vi "Example--SMO.Example.vi"() -> ()   [LabVIEW 2013]
uses:
  SMO.UI.Example/SMO.UI.Example.lvclass
  SMO/Typedefs/SMOState --Enum.ctl
  SMO/Protected/ListThisLevelDependencies.vi
  SMO/reuse/CastArrayDependenciesToClusterOrClass.vi
  SMO.Example/SMO.Example.lvclass
  SMO.UI/SMO.UI.lvclass
  SMO/SMO.lvclass
panel:
  in  "About":bool
  out "Data Changed":string
  out "error out":errorcluster
  in  "Stop":bool
  # "SMO Example Launcher"
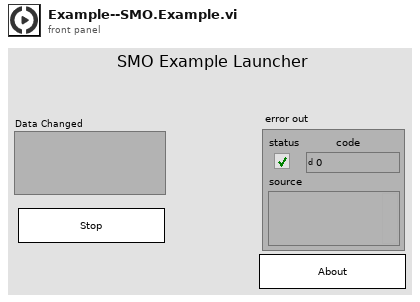
[diagram p1: front panel]
types:
  T1 = typedef "SMO.lvclass/Public Events.ctl" = cluster{"Error":refnum<user-event>, "State":refnum<user-event>}
  T2 = typedef "SMO.UI.Example.lvclass/Dependencies--Cluster.ctl" = cluster{"SMO.Example":refnum<class "SMO.Example.lvclass">}
  T3 = cluster{"SMO.Example Public Events":refnum<event-registration>, "SMO.UI Public Events":refnum<event-registration>, "Event Registration Refnum":refnum<event-registration>}
  T4 = typedef "SMO.lvclass/SMOState --Enum.ctl" = enum16{"unknown", "Created", "Started", "Stopped"}
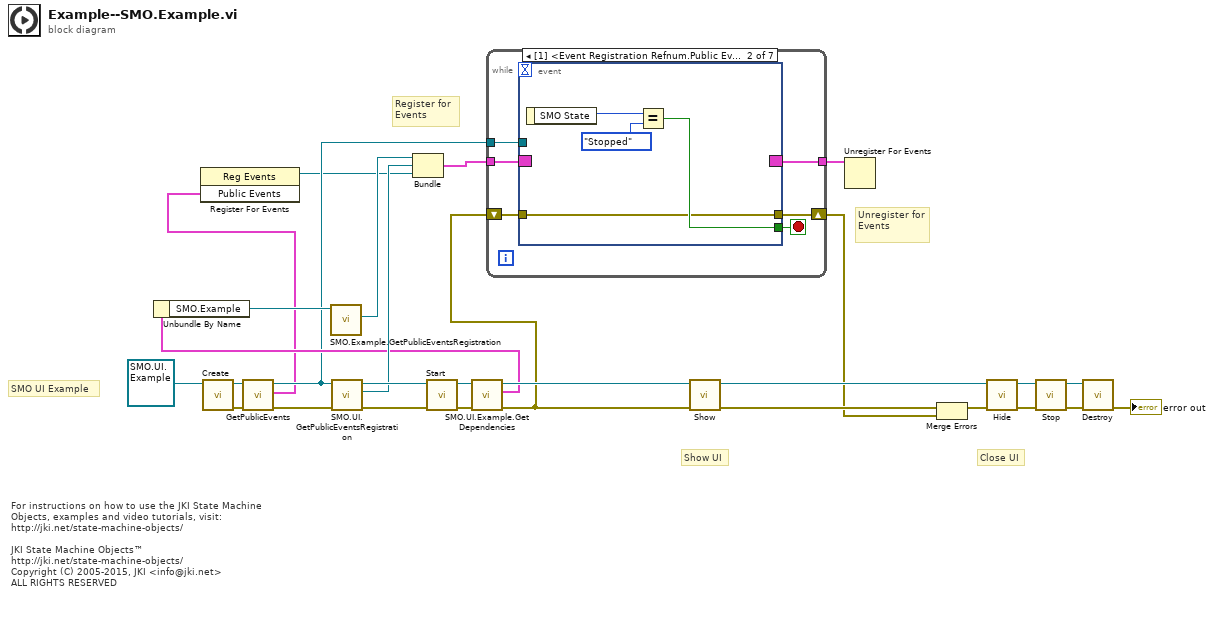
[diagram p0: block diagram]
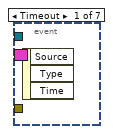
[diagram p2: hidden frame]
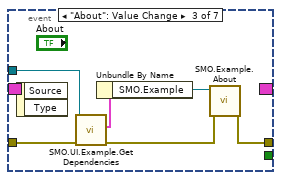
[diagram p3: hidden frame]
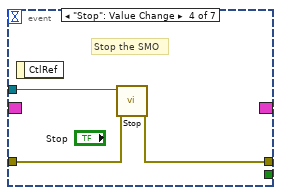
[diagram p4: hidden frame]
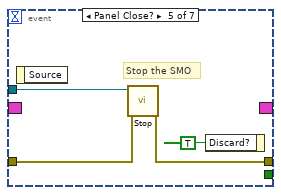
[diagram p5: hidden frame]
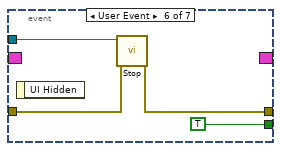
[diagram p6: hidden frame]
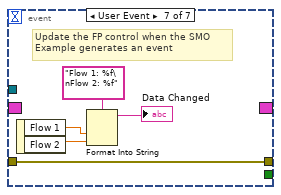
[diagram p7: hidden frame]
diagram:
  # "Close UI"
  # "Show UI"
  # "SMO UI Example"
  # "For instructions on how to use the JKI State Machine Objects, examples and video tutorials, visit:\nhttp://jki.net/state-machine-objects/\n\nJKI State Machine Objects™\nhttp://jki.net/state-machine-objects/\nCopyright (C) 2005-2015, JKI <info@jki.net>\nALL RIGHTS RESERVED"
  # "Unregister for Events"
  # "Register for Events"
  n1 = call "Create.vi"("SMO"=refnum<class "SMO.UI.Example.lvclass"> refnum ("SMO.UI.Example.lvclass")) -> ("error out"=w4:errorcluster, "SMO out"=w6:refnum<class "SMO.UI.Example.lvclass">)  [unwired: 8 in, 1 out]
  n2 = call "GetPublicEvents.vi"("error in (no error)"=w4, "SMO"=w6) -> ("error out"=w3:errorcluster, "Public Events"=w2:T1, "SMO out"=w5:refnum<class "SMO.UI.Example.lvclass">)  [unwired: 7 in]
  n3 = register-events(w2) -> (reference out=w1:refnum<event-registration>)  [unwired: 2 in, 1 out]
  n4 = call "SMO.UI.GetPublicEventsRegistration.vi"("error in (no error)"=w3, "SMO.UI"=w5) -> ("error out"=w23:errorcluster, "SMO.UI Public Events"=w21:refnum<event-registration>, "SMO.UI out"=w22:refnum<class "SMO.UI.Example.lvclass">)  [unwired: 7 in]
  n5 = call "Start.vi"("error in (no error)"=w23, "SMO"=w22) -> ("error out"=w11:errorcluster, "SMO out"=w13:refnum<class "SMO.UI.Example.lvclass">)  [unwired: 8 in]
  n6 = call "SMO.UI.Example.Get Dependencies.vi"("error in (no error)"=w11, "SMO UI.Template in"=w13) -> ("error out"=w8:errorcluster, "Dependencies"=w10:T2, "SMO UI.Template out"=w12:refnum<class "SMO.UI.Example.lvclass">)  [unwired: 7 in]
  n7 = Unbundle By Name(w10) -> ("SMO.Example"=w9:refnum<class "SMO.Example.lvclass">)
  n8 = call "SMO.Example.GetPublicEventsRegistration.vi"("SMO.Example"=w9) -> ("SMO.Example Public Events"=w20:refnum<event-registration>)  [unwired: 8 in, 2 out]
  n9 = Bundle("SMO.Example Public Events"=w20, "SMO.UI Public Events"=w21, "Event Registration Refnum"=w1) -> (w19:T3)  [unwired: 1 in]
  n10 = while {
    tunnel: w5 -> [w33]
    shift-right: [w32] -> w7
    shift-left: w8 -> [w31]
    tunnel: w19 -> [w30]
    tunnel: [w29] -> w28
    stop <- w34 stop-if-true
    n11 = event shown="[1] <Event Registration Refnum.Public Events.State>: User Event" {
      selector: w30 -> [_ _ _ _ _ _ _]
      dyn-events: [_ _ _ _ _ _ _] -> w29
      timeout: _ -> [_ _ _ _ _ _ _]
      tunnel: [_ w36 _ _ _ TRUE ("OK") _] -> w34
      tunnel: w33 -> [_ _ w43 w47 w51 w55 _]
      tunnel: [_ w35 w44 w46 w49 w53 w59] -> w32
      tunnel: w31 -> [_ w35 w42 w45 w48 w54 w59]
      event Timeout {
        n12 = event-data() -> ()  [unwired: 1 in, 3 out]
      }
      event User Event {
        n13 = event-data() -> ("SMO State"=w38:T4)  [unwired: 1 in]
        n14 = Equal?(x=w38, y=SMOState_--Enum."Stopped") -> (x = y?=w36:bool)
      }
      event "About": Value Change {
        n15 = event-data() -> ()  [unwired: 1 in, 2 out]
        n16 = call "SMO.UI.Example.Get Dependencies.vi"("error in (no error)"=w42, "SMO UI.Template in"=w43) -> ("error out"=w41:errorcluster, "Dependencies"=w40:T2)  [unwired: 7 in, 1 out]
        n17 = Unbundle By Name(w40) -> ("SMO.Example"=w39:refnum<class "SMO.Example.lvclass">)
        n18 = call "SMO.Example.About.vi"("error in (no error)"=w41, "SMO.Example"=w39) -> ("error out"=w44:errorcluster)  [unwired: 8 in, 1 out]
      }
      event "Stop": Value Change {
        # "Stop the SMO"
        n19 = event-data() -> ()  [unwired: 1 in, 1 out]
        n20 = call "Stop.vi"("error in (no error)"=w45, "SMO"=w47) -> ("error out"=w46:errorcluster)  [unwired: 8 in, 1 out]
      }
      event Panel Close? {
        # "Stop the SMO"
        n21 = event-data() -> ()  [unwired: 1 in, 1 out]
        n22 = call "Stop.vi"("error in (no error)"=w48, "SMO"=w51) -> ("error out"=w49:errorcluster)  [unwired: 8 in, 1 out]
        n23 = event-data("Discard?"=TRUE ("OK")) -> ()  [unwired: 1 in, 1 out]
      }
      event User Event {
        n24 = event-data() -> ()  [unwired: 1 in, 1 out]
        n25 = call "Stop.vi"("error in (no error)"=w54, "SMO"=w55) -> ("error out"=w53:errorcluster)  [unwired: 8 in, 1 out]
      }
      event User Event {
        # "Update the FP control when the SMO\nExample generates an event"
        n26 = event-data() -> ("Flow 1"=w57:dbl, "Flow 2"=w56:dbl)  [unwired: 1 in]
        n27 = Format Into String(format string="Flow 1: %f\nFlow 2: %f", w57, w56) -> (resulting string=→"Data Changed":string)  [unwired: 2 in, 1 out]
      }
    }
  }
  n28 = call "Show.vi"("error in (no error)"=w8, "SMO.UI"=w12) -> ("error out"=w26:errorcluster, "SMO.UI out"=w14:refnum<class "SMO.UI.Example.lvclass">)  [unwired: 8 in]
  n29 = Unregister For Events(event registration refnum=w28) -> ()  [unwired: 1 in, 1 out]
  n30 = Merge Errors(w26, w7) -> (w25:errorcluster)
  n31 = call "Hide.vi"("error in (no error)"=w25, "SMO.UI"=w14) -> ("error out"=w15:errorcluster, "SMO.UI out"=w18:refnum<class "SMO.UI.Example.lvclass">)  [unwired: 8 in]
  n32 = call "Stop.vi"("error in (no error)"=w15, "SMO"=w18) -> ("error out"=w16:errorcluster, "SMO out"=w17:refnum<class "SMO.UI.Example.lvclass">)  [unwired: 8 in]
  n33 = call "Destroy.vi"("error in (no error)"=w16, "SMO"=w17) -> ("error out"=→"error out":errorcluster)  [unwired: 9 in]
